vi "ma_ParamDesigner.vi"(3 "Desired Filter Specifications":T1 {"PB Gain" format="%0.2f"; "SB Gain" format="%0.2f"; "Lower SB" format="%0.2p"; "Upper SB" format="%0.2f"; "Lower PB" format="%0.2p"; "Upper PB" format="%0.2f"}, 4 "Filter type":T2(ring), 5 "Sampling Frequency":dbl format="%0.2f", 6 "Filter topology":T3(ring)) -> (0 "filter order":i32, 1 "fh":dbl format="%0.2f", 2 "fl":dbl format="%0.2f")   [LabVIEW 2020, in "NI_MAPro.lvlib"]
uses:
  NI_MAPro.lvlib
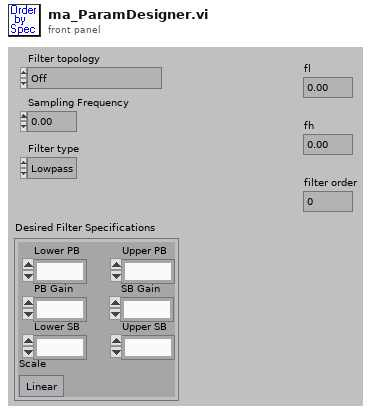
[diagram p1: front panel]
types:
  T1 = cluster{"Lower PB":dbl, "Upper PB":dbl, "Lower SB":dbl, "Upper SB":dbl, "PB Gain":dbl, "SB Gain":dbl, "Scale":bool}
  T2 = enum32{"Lowpass", "Highpass", "Bandpass", "Bandstop"}
  T3 = enum32{"Off", "Butterworth", "Chebyshev", "Inverse Chebyshev", "Elliptic", "Bessel"}
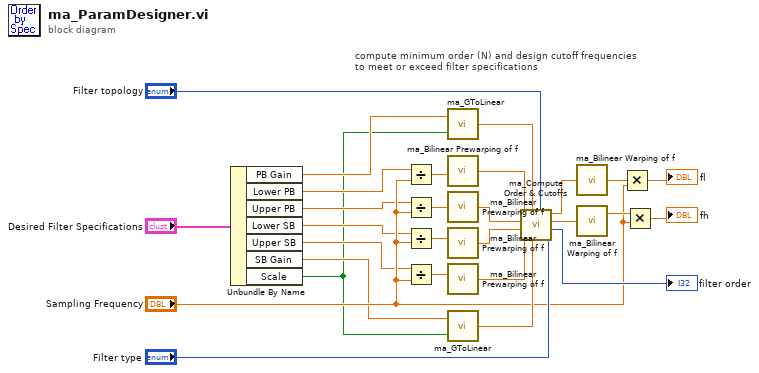
[diagram p0: block diagram]
diagram:
  # "compute minimum order (N) and design cutoff frequencies\nto meet or exceed filter specifications"
  n1 = Unbundle By Name("Desired Filter Specifications") -> ("PB Gain"=w7:dbl, "Lower PB"=w6:dbl, "Upper PB"=w5:dbl, "Lower SB"=w4:dbl, "Upper SB"=w3:dbl, "SB Gain"=w2:dbl, "Scale"=w1:bool)
  n2 = Divide(x=w6, y="Sampling Frequency") -> (x/y=w18:dbl)
  n3 = Divide(x=w5, y="Sampling Frequency") -> (x/y=w19:dbl)
  n4 = Divide(x=w4, y="Sampling Frequency") -> (x/y=w20:dbl)
  n5 = Divide(x=w3, y="Sampling Frequency") -> (x/y=w21:dbl)
  n6 = call "ma_GToLinear.vi"("G unit"=w1, "G"=w7) -> ("G (linear)"=w25:dbl)
  n7 = call "ma_Bilinear Prewarping of f.vi"("f"=w18) -> ("prewarped f"=w12:dbl)
  n8 = call "ma_Bilinear Prewarping of f.vi"("f"=w19) -> ("prewarped f"=w13:dbl)
  n9 = call "ma_Bilinear Prewarping of f.vi"("f"=w20) -> ("prewarped f"=w14:dbl)
  n10 = call "ma_Bilinear Prewarping of f.vi"("f"=w21) -> ("prewarped f"=w15:dbl)
  n11 = call "ma_GToLinear.vi"("G unit"=w1, "G"=w2) -> ("G (linear)"=w24:dbl)
  n12 = call "ma_Compute Order & Cutoffs.vi"("filter type"="Filter type", "filter design"="Filter topology", "Gs"=w24, "Gp"=w25, "fs2"=w15, "fs1"=w14, "fp2"=w13, "fp1"=w12) -> ("N"=→"filter order":i32, "fh"=w17:dbl, "fl"=w16:dbl)
  n13 = call "ma_Bilinear Warping of f.vi"("f"=w16) -> ("prewarped f"=w22:dbl)
  n14 = call "ma_Bilinear Warping of f.vi"("f"=w17) -> ("prewarped f"=w23:dbl)
  n15 = Multiply(x=w22, y="Sampling Frequency") -> (x*y=→"fl":dbl)
  n16 = Multiply(x=w23, y="Sampling Frequency") -> (x*y=→"fh":dbl)
